vi "DrawSubMenuText.vi"(4 "Enable":bool, 6 "ShortcutText":string, 7 "Collection in":refnum<class "Collection.lvclass">, 8 "error in (no error)":errorcluster, 9 "Text":refnum<class "Text.lvclass">, 10 "InsertionPoint":refnum<class "Point.lvclass">, 11 "Menu in":refnum<class "Menu.lvclass">) -> (0 "error out":errorcluster, 3 "Menu out":refnum<class "Menu.lvclass">, 5 "Collection out":refnum<class "Collection.lvclass">)   [LabVIEW 2021, in "Menu.lvlib" / "Menu.lvclass"]
uses:
  Menu.lvclass
  Menu.lvclass/Menu.ctl
  Picture2D/src/Collection/Collection.lvclass
  Picture2D/src/Text/Text.lvclass
  Picture2D/src/Point/Point.lvclass
  C:/GitHub/Picture2D/src/Shape/Shape.lvclass
  C:/GitHub/Picture2D/src/Picture2D/Picture2D.lvclass
  C:/GitHub/Picture2D/src/IDrawable/IDrawable.lvclass
  C:/GitHub/Picture2D/src/IMovable/IMovable.lvclass
  C:/GitHub/Picture2D/src/IRotatable/IRotatable.lvclass
  C:/GitHub/Picture2D/src/IScalable/IScalable.lvclass
  C:/GitHub/Picture2D/src/Text/Text.lvclass
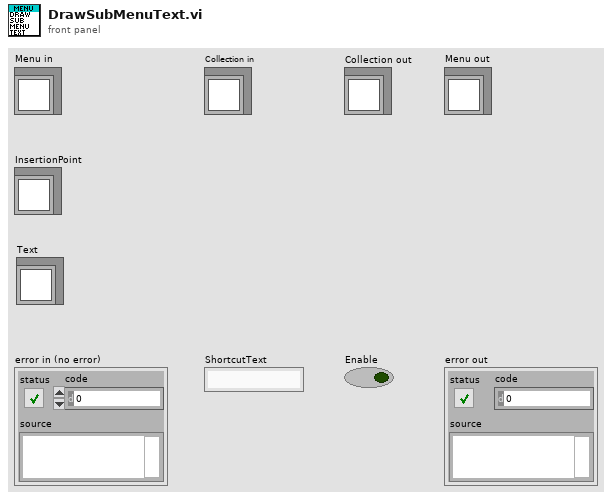
[diagram p1: front panel]
types:
  T1 = enum16{"User-specified Font", "Application Font", "System Font", "Dialog Font"}
  T2 = typedef "Menu.lvlib/Menu.lvclass/MenuColors.ctl" = cluster{"Text":refnum<class "Color.lvclass">, "HiliteText":refnum<class "Color.lvclass">, "Background":refnum<class "Color.lvclass">, "BorderColor":refnum<class "Color.lvclass">, "Hilite":refnum<class "Color.lvclass">}
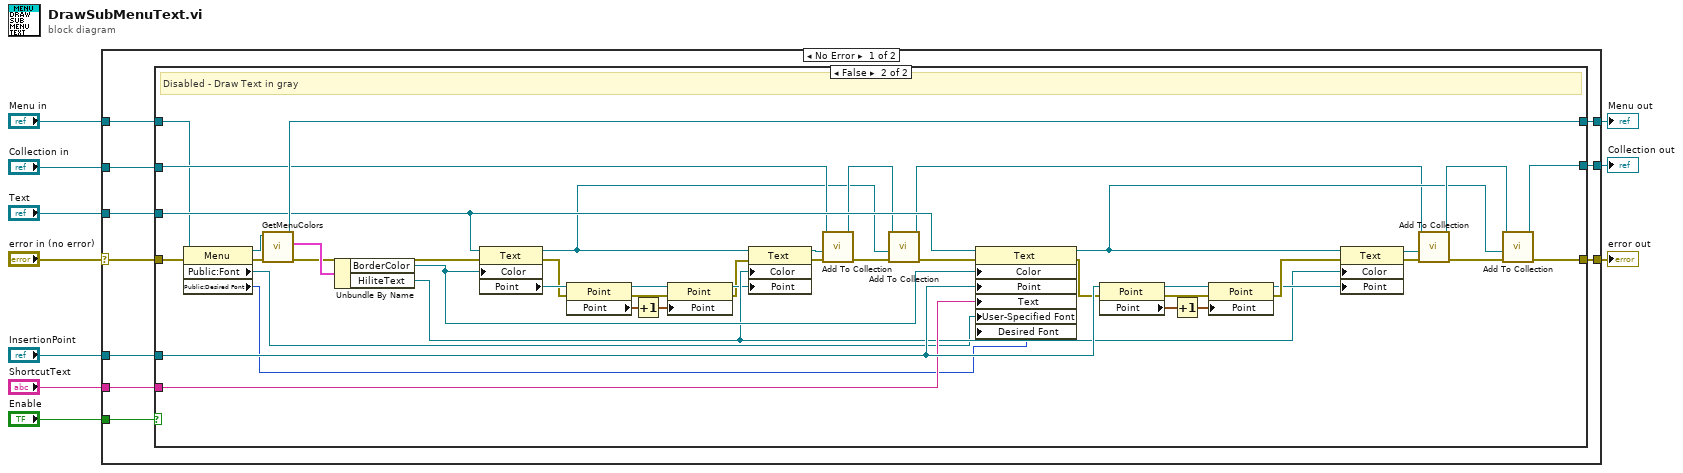
[diagram p0: block diagram]
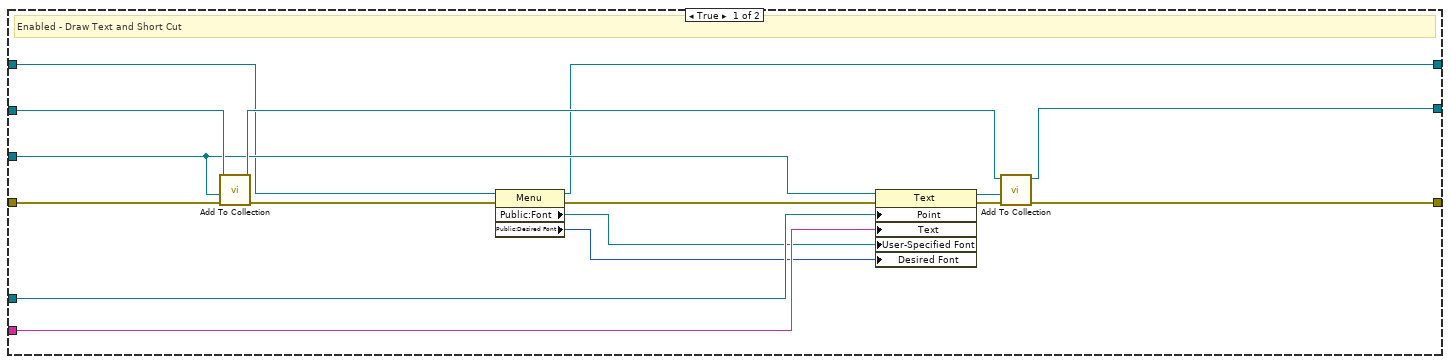
[diagram p2: hidden frame]
diagram:
  n1 = case shown="No Error" "error in (no error)" {
    selector: "error in (no error)" -> [w19 w81]
    tunnel: [w20 w81] -> w10
    tunnel: "InsertionPoint" -> [w18 _]
    tunnel: [w17 w82] -> w7
    tunnel: "ShortcutText" -> [w16 _]
    tunnel: "Text" -> [w15 _]
    tunnel: "Collection in" -> [w14 w82]
    tunnel: "Menu in" -> [w13 w83]
    tunnel: [w12 w83] -> w2
    tunnel: "Enable" -> [w11 _]
    frame No Error {
      n2 = case shown="False" w11 {
        tunnel: [w31 w68] -> w20
        tunnel: w19 -> [w29 w42]
        tunnel: w18 -> [w33 w80]
        tunnel: [w35 w66] -> w17
        tunnel: w16 -> [w34 w79]
        tunnel: w15 -> [w26 w64]
        tunnel: w14 -> [w27 w54]
        tunnel: w13 -> [w24 w41]
        tunnel: [w23 w70] -> w12
        frame True {
          # "Enabled - Draw Text and Short Cut"
          n3 = call-dynamic "Add To Collection.vi"("error in (no error)"=w29, "IDrawable"=w26, "Collection in"=w27) -> ("error out"=w30:errorcluster, "Collection out"=w28:refnum<class "Collection.lvclass">)  [unwired: 7 in]
          n4 = property class="Menu"(reference=w24, error in=w30) -> (reference out=w23:refnum<class "Menu.lvclass">, error out=w25:errorcluster, "Public:Font"=w22:refnum<class "Font.lvclass">, "Public:Desired Font"=w21:T1)
          n5 = property class="Text"(reference=w26, error in=w25, "Point"=w33, "Text"=w34, "User-Specified Font"=w22, "Desired Font"=w21) -> (reference out=w36:refnum<class "Text.lvclass">, error out=w32:errorcluster)
          n6 = call-dynamic "Add To Collection.vi"("error in (no error)"=w32, "IDrawable"=w36, "Collection in"=w28) -> ("error out"=w31:errorcluster, "Collection out"=w35:refnum<class "Collection.lvclass">)  [unwired: 7 in]
        }
        frame False {
          # "Disabled - Draw Text in gray"
          n7 = property class="Menu"(reference=w41, error in=w42) -> (reference out=w39:refnum<class "Menu.lvclass">, error out=w40:errorcluster, "Public:Font"=w38:refnum<class "Font.lvclass">, "Public:Desired Font"=w37:T1)
          n8 = call "GetMenuColors.vi"("error in (no error)"=w40, "Menu in"=w39) -> ("error out"=w60:errorcluster, "MenuColors"=w71:T2, "Menu out"=w70:refnum<class "Menu.lvclass">)  [unwired: 7 in]
          n9 = Unbundle By Name(w71) -> ("BorderColor"=w61:refnum<class "Color.lvclass">, "HiliteText"=w50:refnum<class "Color.lvclass">)
          n10 = property class="Text"(reference=w64, error in=w60, "Color"=w61) -> (reference out=w48:refnum<class "Text.lvclass">, error out=w44:errorcluster, "Point"=w58:refnum<class "Point.lvclass">)
          n11 = property class="Point"(reference=w58, error in=w44) -> (reference out=w57:refnum<class "Point.lvclass">, error out=w56:errorcluster, "Point"=w45:cluster{"x":i16, "y":i16})
          n12 = Increment(x=w45) -> (x+1=w47:cluster{"x":i16, "y":i16})
          n13 = property class="Point"(reference=w57, error in=w56, "Point"=w47) -> (reference out=w49:refnum<class "Point.lvclass">, error out=w43:errorcluster)
          n14 = property class="Text"(reference=w48, error in=w43, "Color"=w50, "Point"=w49) -> (reference out=w52:refnum<class "Text.lvclass">, error out=w51:errorcluster)
          n15 = call-dynamic "Add To Collection.vi"("error in (no error)"=w51, "IDrawable"=w52, "Collection in"=w54) -> ("error out"=w55:errorcluster, "Collection out"=w53:refnum<class "Collection.lvclass">)  [unwired: 7 in]
          n16 = call-dynamic "Add To Collection.vi"("error in (no error)"=w55, "IDrawable"=w48, "Collection in"=w53) -> ("error out"=w62:errorcluster, "Collection out"=w63:refnum<class "Collection.lvclass">)  [unwired: 7 in]
          n17 = property class="Text"(reference=w64, error in=w62, "Color"=w61, "Point"=w80, "Text"=w79, "User-Specified Font"=w38, "Desired Font"=w37) -> (reference out=w65:refnum<class "Text.lvclass">, error out=w74:errorcluster)
          n18 = property class="Point"(reference=w80, error in=w74) -> (reference out=w78:refnum<class "Point.lvclass">, error out=w77:errorcluster, "Point"=w46:cluster{"x":i16, "y":i16})
          n19 = Increment(x=w46) -> (x+1=w59:cluster{"x":i16, "y":i16})
          n20 = property class="Point"(reference=w78, error in=w77, "Point"=w59) -> (reference out=w75:refnum<class "Point.lvclass">, error out=w76:errorcluster)
          n21 = property class="Text"(reference=w65, error in=w76, "Color"=w50, "Point"=w75) -> (reference out=w73:refnum<class "Text.lvclass">, error out=w72:errorcluster)
          n22 = call-dynamic "Add To Collection.vi"("error in (no error)"=w72, "IDrawable"=w73, "Collection in"=w63) -> ("error out"=w69:errorcluster, "Collection out"=w67:refnum<class "Collection.lvclass">)  [unwired: 7 in]
          n23 = call-dynamic "Add To Collection.vi"("error in (no error)"=w69, "IDrawable"=w65, "Collection in"=w67) -> ("error out"=w68:errorcluster, "Collection out"=w66:refnum<class "Collection.lvclass">)  [unwired: 7 in]
        }
      }
    }
    frame Error {
    }
  }
  "error out" <- w10
  "Collection out" <- w7
  "Menu out" <- w2
